vi "Begin.vi"(8 "error in":errorcluster, 11 "Image Size":T6=enum."320x240") -> (0 "error out":errorcluster)   [LabVIEW 2016]
doc: "Called before other user functions, this VI is expected to open initial I/O refnums, load in file data, and do all program initialization. Notice that the <B>error out</B> terminal is simply used for data flow. Wiring it to other structures or subVIs ensures that this VI runs first."
uses:
  <vilib>/Rock Robotics/WPI/RobotDrive/WPI_RobotDriveDevRef.ctl
  <vilib>/Rock Robotics/WPI/MotorControl/WPI_MotorControlDeviceRef.ctl
  <vilib>/Rock Robotics/WPI/MotorControl/WPI_MotorControlType.ctl
  <vilib>/Rock Robotics/SystemInterfaces/DIO/FPGA_DIOPWMChannel.ctl
  <vilib>/Rock Robotics/WPI/PWM/WPI_PWMDeadband.ctl
  <vilib>/Rock Robotics/WPI/Camera/WPI_CameraImageSize.ctl
  <vilib>/Rock Robotics/WPI/DriverStation/WPI_DriverStationRobotMode2.ctl
  <vilib>/Rock Robotics/WPI/Joystick/WPI_JoystickDeviceEnum.ctl
  <vilib>/Rock Robotics/SystemInterfaces/DIO/FPGA_DIOChannel.ctl
  <vilib>/Rock Robotics/SystemInterfaces/AI/FPGA_AIGyroChannel.ctl
  <vilib>/Rock Robotics/WPI/Solenoid/WPI_SolenoidChannel.ctl
  Single Talon.ctl
  <vilib>/Rock Robotics/WPI/ThirdParty/CanMotor/TalonSRX/WPI_CANTalonSRX_APIControlMode.ctl
  <vilib>/Rock Robotics/SystemInterfaces/DIO/FPGA_DIORelayChannel.ctl
  <vilib>/Rock Robotics/WPI/Camera/WPI_CameraWhite Balance Values.ctl
  <vilib>/Rock Robotics/WPI/Camera/WPI_CameraExposure Values.ctl
  <vilib>/Rock Robotics/WPI/Camera/WPI_CameraFrameRate.ctl
  Robot Global Data.vi
  <vilib>/Rock Robotics/Network Tables/NT Write String Array.vi
  <vilib>/Rock Robotics/WPI/Counter/WPI_CounterDigitalInputToDigitalSource.vi
  <vilib>/Rock Robotics/WPI/Gyro/WPI_GyroAnalogOpen.vi
  <vilib>/Rock Robotics/WPI/Ultrasonic/WPI_SonarSRF04DigitalOpen.vi
  <vilib>/Rock Robotics/WPI/Ultrasonic/WPI_SonarSRF04DigitalRefNum Registry Set.vi
  <vilib>/Rock Robotics/WPI/Switch/WPI_SwitchOpenLimit.vi
  <vilib>/Rock Robotics/WPI/RobotDrive/WPI_RobotDriveOpen2MotorWithExistingMotors.vi
  <vilib>/Rock Robotics/WPI/Solenoid/WPI_SolenoidOpenDouble.vi
panel:
  out "Testing DevRef 2":T1={"DevStatus"={"status"=FALSE, "code"=0, "source"=""}, "Motors[]"=[], "Square Inputs"=FALSE, "Max Output"=1.0}
  out "Testing DevRef":T1={"DevStatus"={"status"=FALSE, "code"=0, "source"=""}, "Motors[]"=[], "Square Inputs"=FALSE, "Max Output"=1.0}
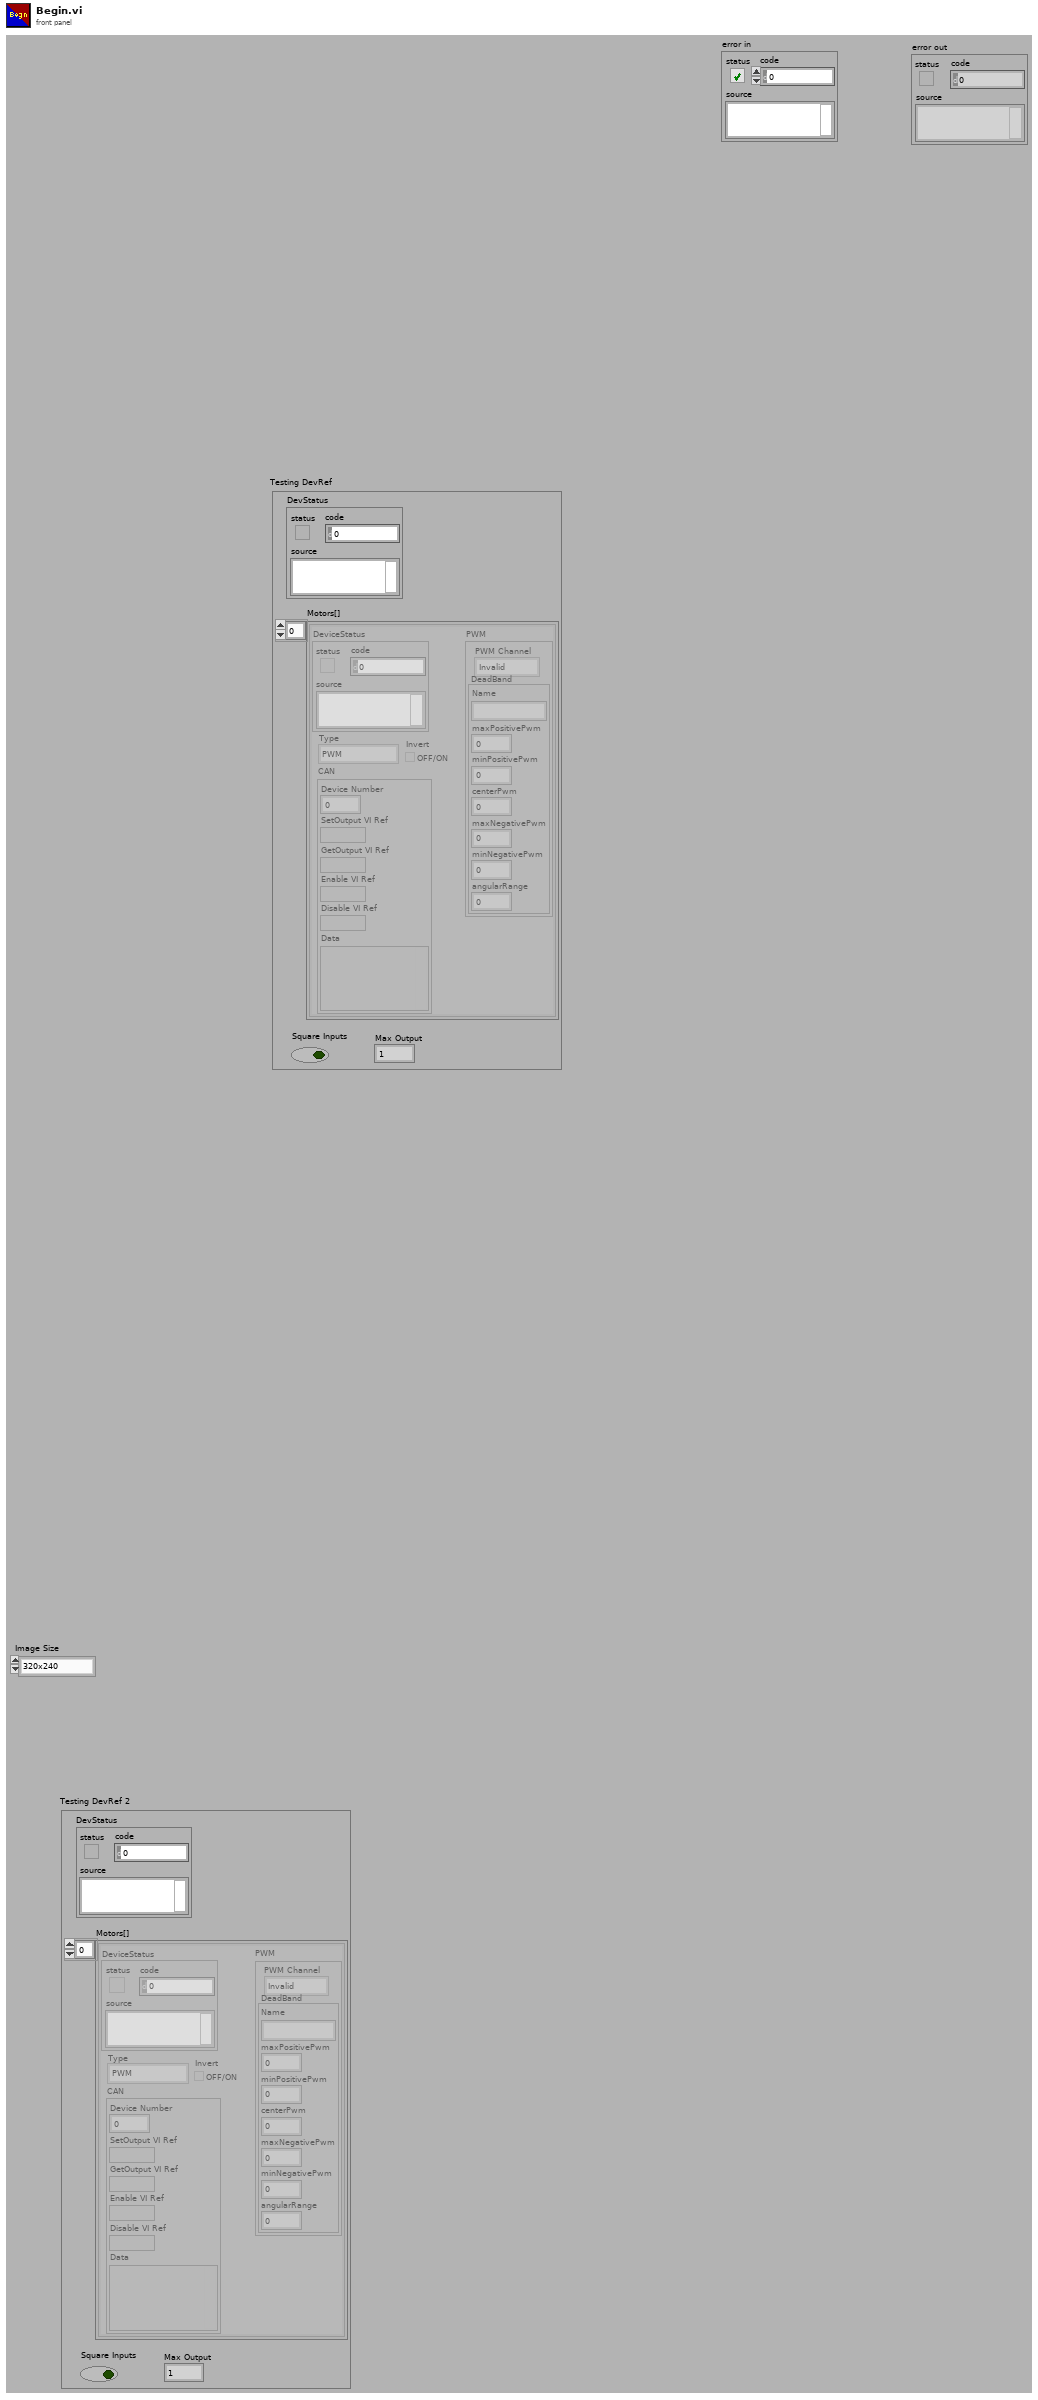
[diagram p1: front panel]
types:
  T1 = typedef "WPI_RobotDriveDevRef.ctl" = cluster{"DevStatus":errorcluster, "Motors[]":T2[], "Square Inputs":bool, "Max Output":dbl}
  T2 = typedef "WPI_MotorControlDeviceRef.ctl" = cluster{"DeviceStatus":errorcluster, "Type":T3, "PWM":cluster{"PWM Channel":T4, "DeadBand":T5}, "CAN":cluster{"Device Number":u8, "SetOutput VI Ref":variant, "GetOutput VI Ref":variant, "Enable VI Ref":variant, "Disable VI Ref":variant, "Data":variant}, "Invert":bool}
  T3 = typedef "WPI_MotorControlType.ctl" = enum16{"PWM", "CAN"}
  T4 = typedef "FPGA_DIOPWMChannel.ctl" = enum8{"PWM 0", "PWM 1", "PWM 2", "PWM 3", "PWM 4", "PWM 5", "PWM 6", "PWM 7", "PWM 8", "PWM 9", "PWM MXP 0", "PWM MXP 1", "PWM MXP 2", "PWM MXP 3", "PWM MXP 4", "PWM MXP 5", "PWM MXP 6", "PWM MXP 7", "PWM MXP 8", "PWM MXP 9", "Invalid"}
  T5 = typedef "WPI_PWMDeadband.ctl" = cluster{"Name":string, "maxPositivePwm":i32, "minPositivePwm":i32, "centerPwm":i32, "maxNegativePwm":i32, "minNegativePwm":i32, "angularRange":u16}
  T6 = typedef "WPI_CameraImageSize.ctl" = enum16{"640x480", "320x240", "160x120", "Custom"}
  T7 = typedef "WPI_CameraFrameRate.ctl" = u32
  T8 = typedef "WPI_CameraExposure Values.ctl" = enum16{"Auto", "Flicker-free 50 Hz", "Flicker-free 60 Hz", "Hold current", "Custom"}
  T9 = typedef "WPI_CameraWhite Balance Values.ctl" = enum16{"Auto", "Fixed indoor", "Fixed outdoor 1", "Fixed outdoor 2", "Fixed fluorescent 1", "Fixed fluorescent 2", "Hold current", "Custom"}
  T10 = typedef "FPGA_DIORelayChannel.ctl" = enum8{"Relay 0", "Relay 1", "Relay 2", "Relay 3", "Invalid"}
  T11 = typedef "Single Talon.ctl" = cluster{"ID":i32, "Master ID":i32, "Control Mode":T12, "Invert?":bool, "Name":string}
  T12 = typedef "WPI_CANTalonSRX_APIControlMode.ctl" = enum8{"Percent VBus", "Speed", "Position", "Slave", "Unchanged / Invalid", "Voltage Compensation", "Current", "Motion Profile", "Motion Magic"}
  T13 = typedef "WPI_SolenoidChannel.ctl" = enum8{"Solenoid 0", "Solenoid 1", "Solenoid 2", "Solenoid 3", "Solenoid 4", "Solenoid 5", "Solenoid 6", "Solenoid 7", "Invalid"}
  T14 = typedef "FPGA_DIOChannel.ctl" = enum8{"DIO 0", "DIO 1", "DIO 2", "DIO 3", "DIO 4", "DIO 5", "DIO 6", "DIO 7", "DIO 8", "DIO 9", "DIO MXP 0", "DIO MXP 1", "DIO MXP 2", "DIO MXP 3", "DIO MXP 4", "DIO MXP 5", "DIO MXP 6", "DIO MXP 7", "DIO MXP 8", "DIO MXP 9", "DIO MXP 10", "DIO MXP 11", "DIO MXP 12", "DIO MXP 13", "DIO MXP 14", "DIO MXP 15", "SPI Port CS1", "SPI Port CS2", "SPI Port CS3", "SPI Port MISO", "SPI Port MOSI", "Invalid"}
  T15 = typedef "FPGA_AIGyroChannel.ctl" = enum8{"AI 0", "AI 1", "Invalid"}
  T16 = typedef "WPI_JoystickDeviceEnum.ctl" = enum16{"USB 0", "USB 1", "USB 2", "USB 3", "USB 4", "USB 5"}
  T17 = typedef "WPI_DriverStationRobotMode2.ctl" = enum16{"Autonomous Disabled", "Autonomous Enabled", "Teleop Disabled", "Teleop Enabled", "Disconnected", "Finish", "Test Disabled", "Test Enabled", "Emergency Stopped"}
  T18 = typedef "WPI_JoystickDevRef.ctl" = cluster{"Device":T16}
  T19 = typedef "WPI_SwitchDevRef.ctl" = cluster{"DevStatus":errorcluster, "DIO Channel":T14, "CntIndex":T20, "Normally Closed":bool}
  T20 = typedef "FPGA_CounterCtrSystemIndex.ctl" = enum8{"Ctr 0", "Ctr 1", "Ctr 2", "Ctr 3", "Ctr 4", "Ctr 5", "Ctr 6", "Ctr 7", "Invalid"}
  T21 = typedef "WPI_RelayDevRef.ctl" = cluster{"DevStatus":errorcluster, "Relay Channel":T10, "Relay Direction":T22}
  T22 = typedef "WPI_RelayDirection.ctl" = enum16{"Both directions", "Forward only", "Reverse only"}
  T23 = typedef "WPI_CameraDevRef.ctl" = cluster{"Camera Address":string, "CameraStatus":errorcluster}
  T24 = typedef "WPI_SolenoidDevRef.ctl" = cluster{"DevStatus":errorcluster, "Pneumatics Control Module":u8, "Forward Solenoid Channel":T13, "Reverse Solenoid Channel":T13}
  T25 = typedef "WPI_UltrasonicDeviceRef.ctl" = cluster{"DevStatus":errorcluster, "Ping Channel":T14, "Echo Channel":T14, "CntIndex":T20}
  T26 = typedef "WPI_GyroDevRef.ctl" = cluster{"DevStatus":errorcluster, "Analog Channel":T27, "Offset":dbl, "Gain (VoltsPerDegree/Second)":dbl, "Gyro Type":enum16{"Analog", "XRS450"}, "Handle":i32, "SPI Bus":T28, "Device Found":bool, "Sample Rate":dbl, "Calibrate On Open":bool}
  T27 = typedef "FPGA_AIChannel.ctl" = enum8{"AI 0", "AI 1", "AI 2", "AI 3", "AI MXP 0", "AI MXP 1", "AI MXP 2", "AI MXP 3", "Invalid"}
  T28 = typedef "spi_bus.ctl" = enum16{"SPI On-Board, CS0", "SPI On-Board, CS1", "SPI On-Board, CS2", "SPI On-Board, CS3", "SPI MXP", "Invalid"}
  T29 = typedef "WPI_DigitalInputDevRef.ctl" = cluster{"DevStatus":errorcluster, "DIO Channel":T14}
  T30 = typedef "FPGA_CounterEncoderSourceConvertionLVSourceType.ctl" = cluster{"DevStatus":errorcluster, "AnalogTriggerMode?":bool, "DigitalMode":cluster{"DIO Channel":T31}, "AnalogTriggerMode":cluster{"AnalogTriggerIndex":T32, "OutputType":T33}}
  T31 = typedef "FPGA_DIODigitalSourceChannel.ctl" = enum8{"DIO 0", "DIO 1", "DIO 2", "DIO 3", "DIO 4", "DIO 5", "DIO 6", "DIO 7", "DIO 8", "DIO 9", "DIO MXP 0", "DIO MXP 1", "DIO MXP 2", "DIO MXP 3", "DIO MXP 4", "DIO MXP 5", "DIO MXP 6", "DIO MXP 7", "DIO MXP 8", "DIO MXP 9", "DIO MXP 10", "DIO MXP 11", "DIO MXP 12", "DIO MXP 13", "DIO MXP 14", "DIO MXP 15", "Disabled"}
  T32 = typedef "FPGA_AnalogTriggerIndex.ctl" = enum8{"Trig 0", "Trig 1", "Trig 2", "Trig 3", "Trig 4", "Trig 5", "Trig 6", "Trig 7", "Invalid"}
  T33 = typedef "FPGA_AnalogTriggerOutType.ctl" = enum16{"InWindow", "TriggerState", "Rising", "Falling"}
  T34 = typedef "WPI_EncoderDevRef.ctl" = cluster{"DevStatus":errorcluster, "EncoderIndex":T35, "CounterIndex":T20, "DistancePerCount":dbl, "Decoding Type":T36}
  T35 = typedef "FPGA_EncoderIdx.ctl" = enum8{"Enc 0", "Enc 1", "Enc 2", "Enc 3", "Enc 4", "Enc 5", "Enc 6", "Enc 7", "Invalid"}
  T36 = typedef "WPI_EncoderType.ctl" = enum16{"1x", "2x", "4x"}
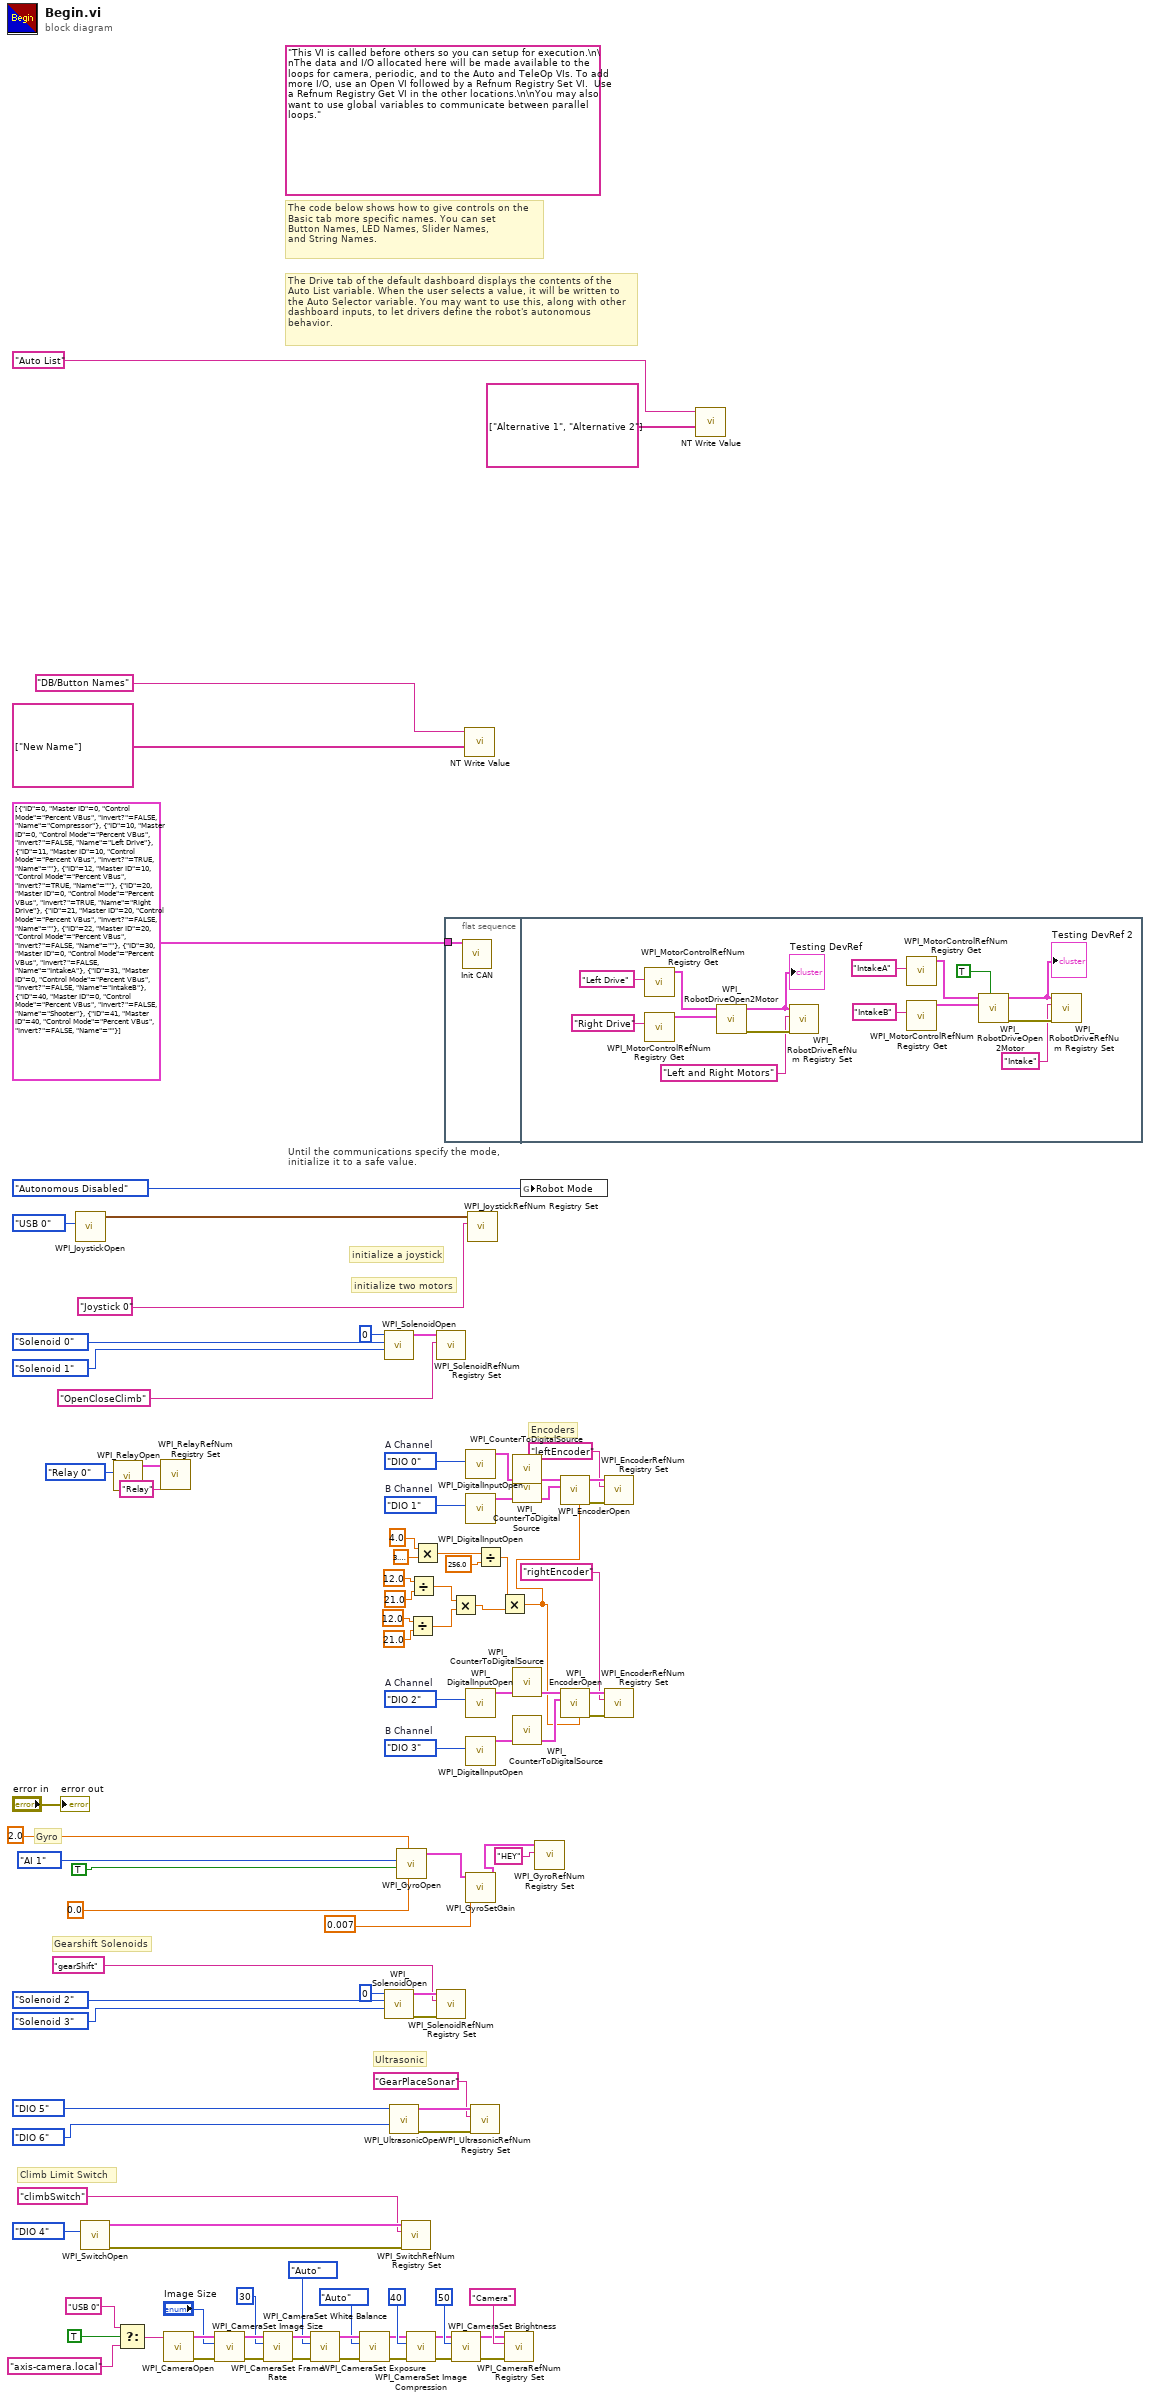
[diagram p0: block diagram]
diagram:
  w79 = FPGA_DIOChannel."DIO 1"  # B Channel
  w78 = FPGA_DIOChannel."DIO 0"  # A Channel
  w88 = FPGA_DIOChannel."DIO 3"  # B Channel
  w87 = FPGA_DIOChannel."DIO 2"  # A Channel
  (unwired) "This VI is called before others so you can setup for execution.\n\nThe data and I/O allocated here will be made available to the loops for camera, periodic, and to the Auto and TeleOp VIs. To add more I/O, use an Open VI followed by a Refnum Registry Set VI.  Use a Refnum Registry Get VI in the other locations.\n\nYou may also want to use global variables to communicate between parallel loops."
  # "Climb Limit Switch"
  # "Ultrasonic"
  # "Gearshift Solenoids"
  # "Encoders"
  # "Gyro"
  # "The Drive tab of the default dashboard displays the contents of the\nAuto List variable. When the user selects a value, it will be written to\nthe Auto Selector variable. You may want to use this, along with other\ndashboard inputs, to let drivers define the robot's autonomous\nbehavior."
  # "The code below shows how to give controls on the\nBasic tab more specific names. You can set\nButton Names, LED Names, Slider Names,\nand String Names."
  # "initialize a joystick"
  # "Until the communications specify the mode,\ninitialize it to a safe value."
  # "initialize two motors"
  n1 = call <vilib>:"WPI_JoystickOpen.vi"("JoystickDevice"=WPI_JoystickDeviceEnum."USB 0") -> ("JoystickDevRef"=w95:T18)  [unwired: 10 in]
  n2 = call-poly <vilib>:"WPI_SwitchOpen.vi"("DIO Channel"=FPGA_DIOChannel."DIO 4") -> ("error out"=w47:errorcluster, "SwitchDevRef"=w46:T19)  [unwired: 9 in]
  n3 = call <vilib>:"WPI_RelayOpen.vi"("Relay Channel"=FPGA_DIORelayChannel."Relay 0") -> ("RelayDevRef"=w35:T21)  [unwired: 9 in, 1 out]
  n4 = Select(t="USB 0" ("format string"), s=TRUE ("dot notation? (F)"), f="axis-camera.local" ("format string")) -> (s? t:f=w10:string)
  n5 = call <vilib>:"WPI_RelayRefNum Registry Set.vi"("refnum name"="Relay", "RelayDevRef"=w35) -> ()  [unwired: 8 in, 2 out]
  n6 = call <vilib>:"WPI_CameraOpen.vi"("Camera Address"=w10) -> ("error out"=w24:errorcluster, "CameraDevRef"=w25:T23)  [unwired: 1 in, 8 out]
  n7 = call <vilib>:"WPI_CameraSet Image Size.vi"("error in (no error)"=w24, "Image Size"="Image Size", "CameraDevRef"=w25) -> ("error out"=w23:errorcluster, "CameraDevRef Out"=w26:T23)  [unwired: 1 in, 6 out]
  n8 = call <vilib>:"WPI_CameraSet Frame Rate.vi"("error in (no error)"=w23, "Frame Rate (fps)"=T7 30, "CameraDevRef"=w26) -> ("error out"=w22:errorcluster, "CameraDevRef Out"=w28:T23)  [unwired: 7 out]
  n9 = call <vilib>:"WPI_CameraSet White Balance.vi"("error in (no error)"=w22, "White Balance"=WPI_CameraWhite_Balance_Values."Auto", "CameraDevRef"=w28) -> ("error out"=w21:errorcluster, "CameraDevRef Out"=w27:T23)  [unwired: 1 in, 6 out]
  n10 = call <vilib>:"WPI_CameraSet Exposure.vi"("error in (no error)"=w21, "Exposure"=WPI_CameraExposure_Values."Auto", "CameraDevRef"=w27) -> ("error out"=w20:errorcluster, "CameraDevRef Out"=w30:T23)  [unwired: 1 in, 6 out]
  n11 = call-poly <vilib>:"WPI_SolenoidOpen.vi"("Reverse Solenoid Channel"=WPI_SolenoidChannel."Solenoid 1", "Forward Solenoid Channel"=WPI_SolenoidChannel."Solenoid 0", "Pneumatics Control Module (0)"=u8 0) -> ("SolenoidDevRef"=w42:T24)  [unwired: 7 in, 1 out]
  n12 = call-poly <vilib>:"WPI_SolenoidOpen.vi"("Reverse Solenoid Channel"=WPI_SolenoidChannel."Solenoid 3", "Forward Solenoid Channel"=WPI_SolenoidChannel."Solenoid 2" ("Solenoid Channel"), "Pneumatics Control Module (0)"=u8 0) -> ("error out"=w55:errorcluster, "SolenoidDevRef"=w56:T24)  [unwired: 7 in]
  n13 = call-poly <vilib>:"WPI_UltrasonicOpen.vi"("Echo DIO Channel"=FPGA_DIOChannel."DIO 6", "Ping DIO Channel"=FPGA_DIOChannel."DIO 5") -> ("error out"=w51:errorcluster, "SonarSRF04DevRef"=w50:T25)  [unwired: 8 in]
  n14 = call-poly <vilib>:"WPI_GyroOpen.vi"("Calibrated Center Voltage"=0.0, "Calibration Time (s)"=2.0, "Calibrate On Open"=TRUE, "Analog Channel"=FPGA_AIGyroChannel."AI 1") -> ("GyroDevRef"=w8:T26)  [unwired: 5 in, 2 out]
  n15 = call <vilib>:"WPI_SwitchRefNum Registry Set.vi"("error in (no error)"=w47, "refnum name"="climbSwitch", "SwitchDevRef"=w46) -> ()  [unwired: 7 in, 2 out]
  n16 = call <vilib>:"WPI_CameraSet Image Compression.vi"("error in (no error)"=w20, "Compression"=40, "CameraDevRef"=w30) -> ("error out"=w19:errorcluster, "CameraDevRef Out"=w29:T23)  [unwired: 7 out]
  n17 = Divide(x=12.0, y=21.0) -> (x/y=w2:dbl)
  n18 = Divide(x=12.0, y=21.0) -> (x/y=w3:dbl)
  n19 = Multiply(x=4.0, y=3.141592653589793) -> (x*y=w68:dbl)
  n20 = call <vilib>:"WPI_SolenoidRefNum Registry Set.vi"("refnum name"="OpenCloseClimb", "SolenoidDevRef"=w42) -> ()  [unwired: 8 in, 2 out]
  n21 = call <vilib>:"WPI_SolenoidRefNum Registry Set.vi"("error in (no error)"=w55, "refnum name"="gearShift", "SolenoidDevRef"=w56) -> ()  [unwired: 7 in, 2 out]
  n22 = flat-sequence {
    tunnel: T11[] [{"ID"=0, "Master ID"=0, "Control Mode"=enum."Percent VBus", "Invert?"=FALSE, "Name"="Compressor"}, {"ID"=10, "Master ID"=0, "Control Mode"=enum."Percent VBus", "Invert?"=FALSE, "Name"="Left Drive"}, {"ID"=11, "Master ID"=10, "Control Mode"=enum."Percent VBus", "Invert?"=TRUE, "Name"=""}, {"ID"=12, "Master ID"=10, "Control Mode"=enum."Percent VBus", "Invert?"=TRUE, "Name"=""}, {"ID"=20, "Master ID"=0, "Control Mode"=enum."Percent VBus", "Invert?"=TRUE, "Name"="Right Drive"}, {"ID"=21, "Master ID"=20, "Control Mode"=enum."Percent VBus", "Invert?"=FALSE, "Name"=""}, {"ID"=22, "Master ID"=20, "Control Mode"=enum."Percent VBus", "Invert?"=FALSE, "Name"=""}, {"ID"=30, "Master ID"=0, "Control Mode"=enum."Percent VBus", "Invert?"=FALSE, "Name"="IntakeA"}, {"ID"=31, "Master ID"=0, "Control Mode"=enum."Percent VBus", "Invert?"=FALSE, "Name"="IntakeB"}, {"ID"=40, "Master ID"=0, "Control Mode"=enum."Percent VBus", "Invert?"=FALSE, "Name"="Shooter"}, {"ID"=41, "Master ID"=40, "Control Mode"=enum."Percent VBus", "Invert?"=FALSE, "Name"=""}] -> [w98]
    frame #0 {
      n23 = call "Init CAN.vi"("Configuration Array"=w98) -> ()  [unwired: 15 in]
    }
    frame #1 {
      n24 = call <vilib>:"WPI_MotorControlRefNum Registry Get.vi"("refnum name"="Left Drive") -> ("MotorControlDevRef"=w113:T2)  [unwired: 9 in, 1 out]
      n25 = call <vilib>:"WPI_MotorControlRefNum Registry Get.vi"("refnum name"="Right Drive") -> ("MotorControlDevRef"=w112:T2)  [unwired: 9 in, 1 out]
      n26 = call-poly <vilib>:"WPI_RobotDriveOpen2Motor.vi"("Right Motor Dev Ref"=w112, "Left Motor Dev Ref"=w113) -> ("error out"=w109:errorcluster, "RobotDriveDevRef"=w108:T1)  [unwired: 8 in]
      "Testing DevRef" <- w108
      n27 = call <vilib>:"WPI_RobotDriveRefNum Registry Set.vi"("error in (no error)"=w109, "refnum name"="Left and Right Motors", "RobotDriveDevRef"=w108) -> ()  [unwired: 7 in, 2 out]
      n28 = call <vilib>:"WPI_MotorControlRefNum Registry Get.vi"("refnum name"="IntakeA") -> ("MotorControlDevRef"=w106:T2)  [unwired: 9 in, 1 out]
      n29 = call <vilib>:"WPI_MotorControlRefNum Registry Get.vi"("refnum name"="IntakeB") -> ("MotorControlDevRef"=w105:T2)  [unwired: 9 in, 1 out]
      n30 = call-poly <vilib>:"WPI_RobotDriveOpen2Motor.vi"("Square Inputs"=TRUE, "Right Motor Dev Ref"=w105, "Left Motor Dev Ref"=w106) -> ("error out"=w102:errorcluster, "RobotDriveDevRef"=w101:T1)  [unwired: 7 in]
      "Testing DevRef 2" <- w101
      n31 = call <vilib>:"WPI_RobotDriveRefNum Registry Set.vi"("error in (no error)"=w102, "refnum name"="Intake", "RobotDriveDevRef"=w101) -> ()  [unwired: 7 in, 2 out]
    }
  }
  n32 = Multiply(x=w3, y=w2) -> (x*y=w1:dbl)
  n33 = call <vilib>:"WPI_CameraSet Brightness.vi"("error in (no error)"=w19, "Brightness"=50, "CameraDevRef"=w29) -> ("error out"=w17:errorcluster, "CameraDevRef Out"=w18:T23)  [unwired: 7 out]
  n34 = call-poly <vilib>:"NT Write Value.vi"("String Array"=string[] ["New Name"], "Name"="DB/Button Names") -> ()  [unwired: 9 in, 1 out]
  n35 = call <vilib>:"WPI_DigitalInputOpen.vi"("DIO Channel"=w78) -> ("DigitalInputDevRef"=w75:T29)  [unwired: 1 in, 9 out]
  n36 = call <vilib>:"WPI_DigitalInputOpen.vi"("DIO Channel"=w79) -> ("DigitalInputDevRef"=w76:T29)  [unwired: 1 in, 9 out]
  n37 = call <vilib>:"WPI_DigitalInputOpen.vi"("DIO Channel"=w87) -> ("DigitalInputDevRef"=w84:T29)  [unwired: 1 in, 9 out]
  n38 = call <vilib>:"WPI_DigitalInputOpen.vi"("DIO Channel"=w88) -> ("DigitalInputDevRef"=w85:T29)  [unwired: 1 in, 9 out]
  n39 = call <vilib>:"WPI_GyroSetGain.vi"("Gain (VoltsPerDegree/Second)"=0.007, "GyroDevRef"=w8) -> ("GyroDevRef"=w7:T26)  [unwired: 8 in, 1 out]
  n40 = call <vilib>:"WPI_JoystickRefNum Registry Set.vi"("refnum name"="Joystick 0", "JoystickDevRef"=w95) -> ()  [unwired: 8 in, 2 out]
  n41 = call-poly <vilib>:"WPI_UltrasonicRefNum Registry Set.vi"("error in (no error)"=w51, "refnum name"="GearPlaceSonar", "SonarSRF04DevRef"=w50) -> ()  [unwired: 7 in, 2 out]
  n42 = Divide(x=w68, y=256.0) -> (x/y=w64:dbl)
  n43 = Multiply(x=w64, y=w1) -> (x*y=w63:dbl)
  n44 = call <vilib>:"WPI_CameraRefNum Registry Set.vi"("error in (no error)"=w17, "refnum name"="Camera", "CameraDevRef"=w18) -> ()  [unwired: 1 in, 8 out]
  n45 = call-poly <vilib>:"WPI_CounterToDigitalSource.vi"("DigitalInputDevRef"=w75) -> ("Digital Source"=w74:T30)  [unwired: 6 out]
  n46 = call-poly <vilib>:"WPI_CounterToDigitalSource.vi"("DigitalInputDevRef"=w76) -> ("Digital Source"=w77:T30)  [unwired: 6 out]
  n47 = call-poly <vilib>:"WPI_CounterToDigitalSource.vi"("DigitalInputDevRef"=w84) -> ("Digital Source"=w83:T30)  [unwired: 6 out]
  n48 = call-poly <vilib>:"WPI_CounterToDigitalSource.vi"("DigitalInputDevRef"=w85) -> ("Digital Source"=w86:T30)  [unwired: 6 out]
  n49 = global write "Robot Global Data.vi" "Robot Mode"(WPI_DriverStationRobotMode2."Autonomous Disabled" ("Robot Mode")) -> ()
  n50 = call <vilib>:"WPI_GyroRefNum Registry Set.vi"("refnum name"="HEY", "GyroDevRef"=w7) -> ()  [unwired: 8 in, 2 out]
  n51 = call <vilib>:"WPI_EncoderOpen.vi"("DistancePerCount"=w63, "BSource"=w77, "ASource"=w74) -> ("error out"=w73:errorcluster, "EncoderDevRef"=w72:T34)  [unwired: 5 in, 2 out]
  n52 = call <vilib>:"WPI_EncoderOpen.vi"("DistancePerCount"=w63, "BSource"=w86, "ASource"=w83) -> ("error out"=w82:errorcluster, "EncoderDevRef"=w81:T34)  [unwired: 5 in, 2 out]
  n53 = call <vilib>:"WPI_EncoderRefNum Registry Set.vi"("error in (no error)"=w73, "refnum name"="leftEncoder", "EncoderDevRef"=w72) -> ()  [unwired: 7 in, 2 out]
  n54 = call <vilib>:"WPI_EncoderRefNum Registry Set.vi"("error in (no error)"=w82, "refnum name"="rightEncoder", "EncoderDevRef"=w81) -> ()  [unwired: 7 in, 2 out]
  n55 = call-poly <vilib>:"NT Write Value.vi"("String Array"=string[] ["Alternative 1", "Alternative 2"], "Name"="Auto List") -> ()  [unwired: 9 in, 1 out]
  "error out" <- "error in"
